vi "RealSense_HelloWorld_PointCloud.vi"() -> ()   [LabVIEW 2017]
doc: "Simple Demo showing how to connect a RealSense Camera to stream COLOR and DEPTH from the stereo camera of a D4xx series camera."
uses:
  libRealSense3.lvlib
  <vilib>/picture/3D Picture Control/NI_3D Picture Control.lvlib
  <vilib>/Utility/miscctls.llb/LV3DPointTypeDef.ctl
  <vilib>/Utility/miscctls.llb/LVRGBAColorTypeDef.ctl
  <vilib>/picture/3D Picture Control/Object/Create Object (name).vi
panel:
  in  "stop and exit":bool
  in  "Color format":enum16{"Monochrome", "RGB internal (RGB)"}(ring)=enum."RGB internal (RGB)"
  in  "Display tab":T1(tab)
  out "Stream selection":u16(ring) items=["Depth + Left Color", "Unrectified L + R", "Rectified L + R", "Depth Only", "RGB ext. Only", "Depth + L Monochrome"]
  out "Found \nRealSense":bool=TRUE
  out "height":i32=720
  out "width":i32=1280
  out "init results":T2={"camera name"="Intel RealSense D415", "camera S/N"="725112060291", "F/W"="05.12.01.00", "Sensor name"="Stereo Module", "api_version"=23201, "rscontext"=2279652045952, "device_list"=2279390748064, "device count"=1, "Dev out"=2279652602464, "sensor_list"=2279759543328, "sensor count"=2, "Sensor out"=2279397784752}
  in  "Select Resolution":u16(ring)=32 items=["424 x 240 @6fps", "424 x 240 @15fps", "424 x 240 @30fps", "424 x 240 @60fps", "424 x 240 @90fps", "480 x 270 @6fps", "480 x 270 @15fps", "480 x 270 @30fps", "480 x 270 @60fps", "480 x 270 @90fps", "640 x 360 @6fps", "640 x 360 @15fps", "640 x 360 @30fps", "640 x 360 @60fps", "640 x 360 @90fps", "640 x 480 @6fps", "640 x 480 @15fps", "640 x 480 @30fps", "640 x 480 @60fps", "640 x 480 @90fps", "848 x 100 @6fps", "848 x 100 @15fps", "848 x 100 @30fps", "848 x 100 @60fps", "848 x 100 @90fps", "848 x 480 @6fps", "848 x 480 @15fps", "848 x 480 @30fps", "848 x 480 @60fps", "848 x 480 @90fps", "1280 x 720 @6fps", "1280 x 720 @15fps", "1280 x 720 @30fps", "1280 x 720 @60fps"]
  in  "Sensor index":i32
  in  "Device index":i32
  out "L-R Baseline, mm":sgl=-54.83181
  out "fy":sgl=952.6064 format="%#_5g"
  out "fx":sgl=952.6064 format="%#_5g"
  out "ppy":sgl=370.69974 format="%#_5g"
  out "ppx":sgl=634.5728 format="%#_5g"
  in  "Exposure,us":sgl=33000.0
  in  "Autoexposure":bool=TRUE
  in  "Depth Presets":T3(ring)=enum."Face2"
  in  "Color Presets":T4(ring)=enum."DS410 (DS5a) 4"
  in  "Laser on/off":bool=TRUE
  in  "Gain(16-248)":sgl=16.0 min=16 max=248
  in  "Update Presets":bool
  in  "Laser \nPower (mW)":dbl(slide)=155.72448 min=0.0 max=360.0 scale=0.36..360.0
  in  "Range Scale":enum16{"200m", "100m", "60m", "6m", "2m", "1m"}(ring)=enum."6m"
  out "RGB image":picture
  out "Depth map":sgl[][](graph)
  out "3D Picture":refnum<vi>(3d-picture)
  out "init error":string="\rNo Error\rNo Error\rNo Error\rNo Error\rNo Error\rNo Error\rNo Error\r\rNo Error\rNo Error"
  out "Capture2 error":string="No Error"
  out "Start Error":string="No Error\rNo Error\rNo Error"
  out "Config error":string="No Error\rNo Error"
  out "Capture1 Error":string="No Error"
  out "Close Error":string="No Error\rNo Error\rNo Error\rNo Error"
  out "release frame error":string="No Error"
  out "iteration":i32=187
  in  "stop":bool=TRUE
  # "RealSense Hello World: PointCloud"
  # "This demo shows how to connect a RealSense D4xx(e) Depth Camera, and display the textured PointCloud."
  # "Note; When you change Depth Preset you need to stop and restart for the HDAD settings to take effect.\n\nTry the Color preset called \"Remove IR2\". It will remove the laser projector from the RGB 1280x720 image."
  # "INTRINSICS & EXTRINSICS"
  # "SELECT THE RESOLUTION"
  # "Recommendation:\nFor D435: 848x480, D415: 1280x720"
  # "COLOR / LEFT MONO"
  # "DEPTH MAP"
  # "Changes Color scale for Depth Map."
  # "20-1660000"
  # "3D POINTCLOUD"
  # "Rotate: Drag image\nMove X-Y: HOLD DOWN CTRL while dragging.\nZoom: SHIFT while dragging."
  # "ERRORS"
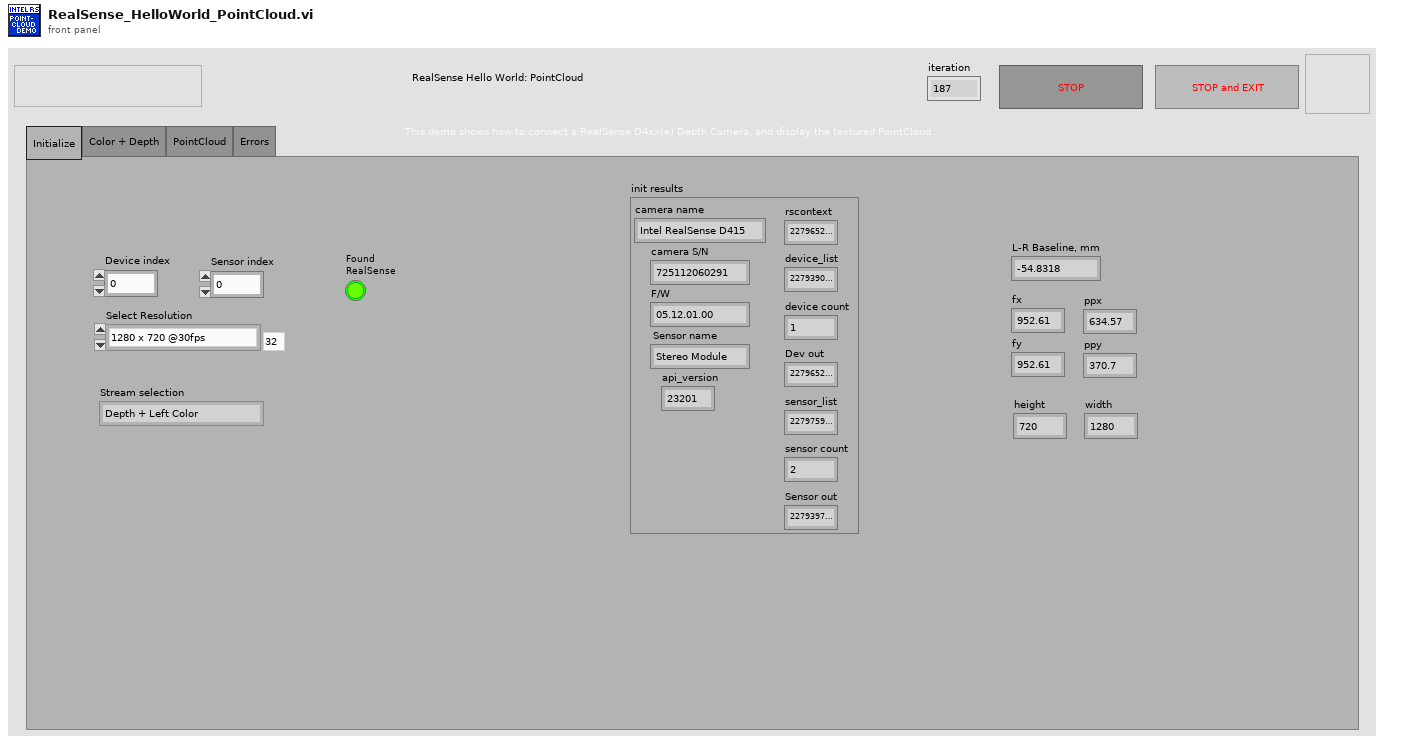
[diagram p1: front panel]
types:
  T1 = enum32{"Initialize", "Color + Depth", "PointCloud", "Errors"}
  T2 = cluster{"camera name":string, "camera S/N":string, "F/W":string, "Sensor name":string, "api_version":i32, "rscontext":u64, "device_list":u64, "device count":i32, "Dev out":u64, "sensor_list":u64, "sensor count":i32, "Sensor out":u64}
  T3 = enum16{"Custom", "Original", "New Depth 1", "New Depth 2", "Depth Active 1", "Active 3D Scan", "Active Short A", "Active Short C", "Face", "Face2", "Best Box", "High Density", "Medium Density", "High Accuracy", "Hand", "Short Range", "Flat wall", "Load .JSON", "Load .JSON2"}
  T4 = enum16{"Custom", "RS400 (DS5p)", "RS400 (DS5p) 2", "RS400 (DS5p) 3", "RS400 (DS5p) 4", "RS400 (DS5p) 5", "RS410 (DS5a)", "RS410 (DS5a) 2", "DS410 (DS5a) 3", "DS410 (DS5a) 4", "DS410+IR", "DS5LR", "DS5LR-2", "DS5LR no pattern", "RS410 Remove IR", "RS410 Remove IR 2", "DS5micro", "D435"}
  T5 = cluster{"width":i32, "height":i32, "fps":i32, "Profile":u64, "ppx":sgl, "ppy":sgl, "fx":sgl, "fy":sgl, "model":u32}
  T6 = enum16{"Overall", "Per Primitive", "Per Vertex", "Binding Off"}
  T7 = enum16{"Points", "Lines", "Line Strip", "Line Loop", "Triangles", "Triangle Strip", "Triangle Fan", "Quads", "Quad Strip", "Polygon"}
  T8 = enum16{"Depth", "Color (ext.)", "Color (left) ", "IR Left", "IR Right", "IR Left (Y16)", "IR Right (Y16)"}
  T9 = cluster{"R":dbl, "G":dbl, "B":dbl, "Alpha":dbl}[]
  T10 = typedef "LVRGBAColorTypeDef.ctl" = cluster{"Red":sgl, "Green":sgl, "Blue":sgl, "Alpha":sgl}
  T11 = typedef "LV3DPointTypeDef.ctl" = cluster{"X":sgl, "Y":sgl, "Z":sgl}
  T12 = cluster{"Alpha":sgl, "Blue":sgl, "Green":sgl, "Red":sgl}
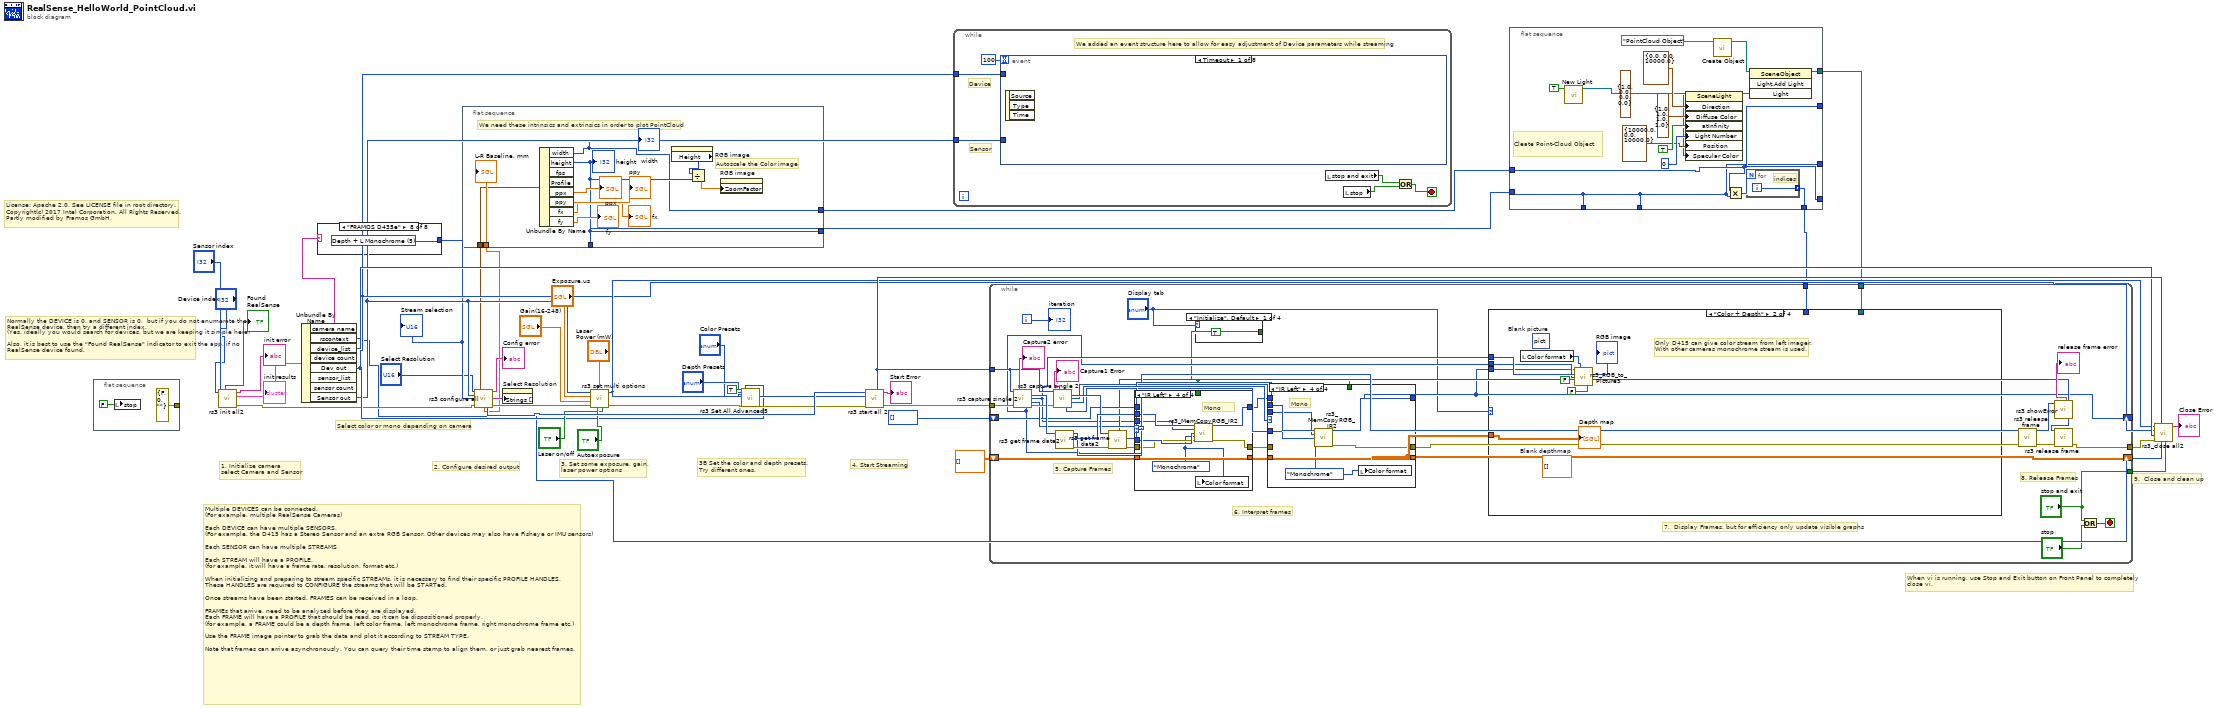
[diagram p0: block diagram]
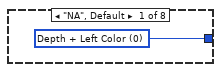
[diagram p2: hidden frame]
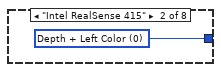
[diagram p3: hidden frame]
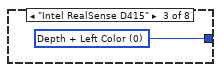
[diagram p4: hidden frame]
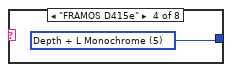
[diagram p5: hidden frame]
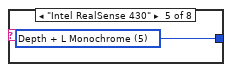
[diagram p6: hidden frame]
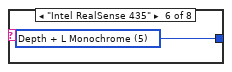
[diagram p7: hidden frame]
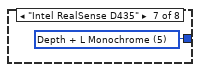
[diagram p8: hidden frame]
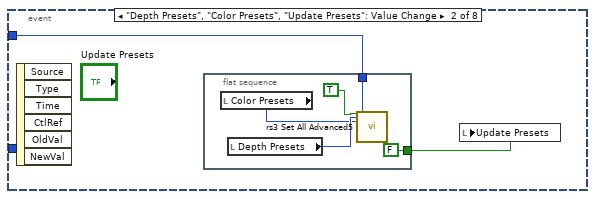
[diagram p9: hidden frame]
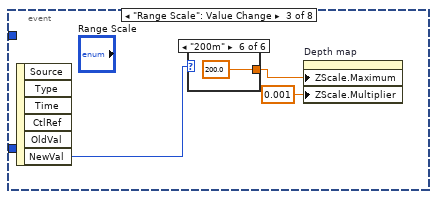
[diagram p10: hidden frame]
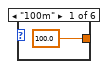
[diagram p11: hidden frame]
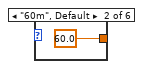
[diagram p12: hidden frame]
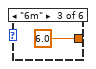
[diagram p13: hidden frame]
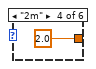
[diagram p14: hidden frame]
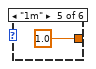
[diagram p15: hidden frame]
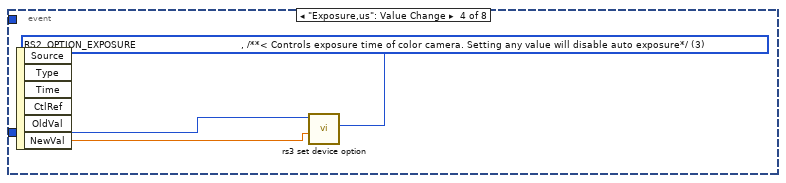
[diagram p16: hidden frame]
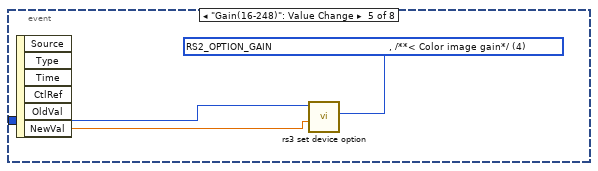
[diagram p17: hidden frame]
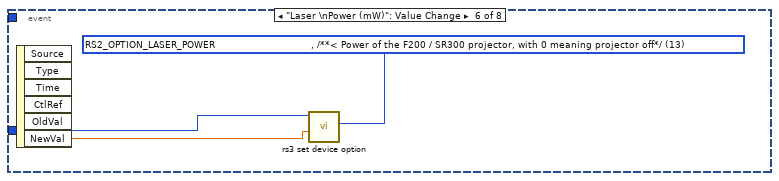
[diagram p18: hidden frame]
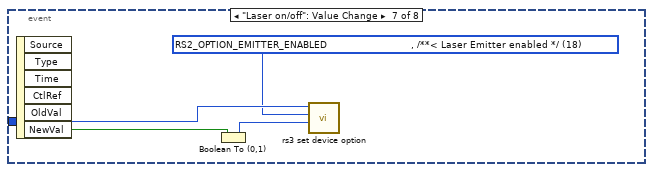
[diagram p19: hidden frame]
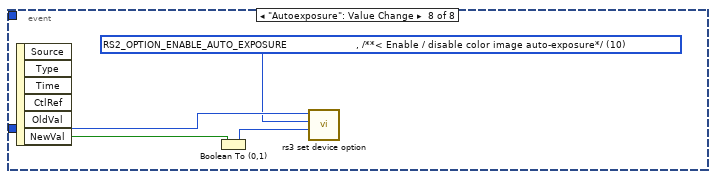
[diagram p20: hidden frame]
diagram:
  # "When vi is running, use Stop and Exit button on Front Panel to completely\nclose vi."
  # "License: Apache 2.0. See LICENSE file in root directory.\nCopyright(c) 2017 Intel Corporation. All Rights Reserved.\nPartly modified by Framos GmbH."
  # "3B Set the color and depth presets.\nTry different ones."
  # "Select color or mono depending on camera"
  # "Normally the DEVICE is 0, and SENSOR is 0,  but if you do not enumerate the RealSense device, then try a different index.\n(Yes, ideally you would search for devices, but we are keeping it simple here)\n\nAlso, it is best to use the \"Found RealSense\" indicator to exit the app, if no RealSense device found."
  # "Multiple DEVICES can be connected. \n(For example, multiple RealSense Cameras)\n\nEach DEVICE can have multiple SENSORS. \n(For example, the D415 has a Stereo Sensor and an extra RGB Sensor. Other devices may also have Fisheye or IMU sensors) \n\nEach SENSOR can have multiple STREAMS\n\nEach STREAM will have a PROFILE. \n(for example, it will have a frame rate, resolution, format etc.)\n\nWhen initializing and preparing to stream specific STREAMs, it is necessary to find their specific PROFILE HANDLES.\nThese HANDLES are required to CONFIGURE the streams that will be STARTed. \n\nOnce streams have been started, FRAMES can be received in a loop. \n \nFRAMEs that arrive, need to be analyzed before they are displayed. \nEach FRAME will have a PROFILE that should be read, so it can be dispositioned properly.\n(for example, a FRAME could be a depth frame, left color frame, left monochrome frame, right monochrome frame etc.)\n\nUse the FRAME image pointer to grab the data and plot it according to STREAM TYPE.\n\nNote that frames can arrive asynchronously. You can query their time stamp to align them, or just grab nearest frames."
  # "9.  Close and clean up"
  # "4. Start Streaming"
  # "3. Set some exposure, gain, \nlaser power options"
  # "2. Configure desired output"
  # "1. Initialize camera\nselect Camera and Sensor"
  n1 = flat-sequence {
    tunnel: [errorcluster {"status"=FALSE, "code"=0, "source"=""} ("error in")] -> _
    frame #0 {
      n2 = local write "stop"(FALSE ("stop")) -> ()
    }
  }
  n3 = call "rs3 init all2.vi"("Select Device"="Device index", "Select Sensor"="Sensor index") -> ("error out"=w9:errorcluster, "init results"=w14:T2, "init error"=→"init error":string, "Found RealSense"=→"Found \nRealSense":bool)  [unwired: 3 in, 3 out]
  "init results" <- w14
  n4 = Unbundle By Name(w14) -> ("camera name"=w8:string, "rscontext"=w6:u64, "device_list"=w37:u64, "Dev out"=w21:u64, "Sensor out"=w20:u64)  [unwired: 3 out]
  n5 = case shown="\"FRAMOS D435e\"" w8 {
    tunnel: [w45 w46 w47 w48 w49 w50 w51 w52] -> w7
    frame "NA", Default {
      w45 = u16 0 items=["Depth + Left Color", "Unrectified L + R", "Rectified L + R", "Depth Only", "RGB ext. Only", "Depth + L Monochrome"] ("Stream selection")
    }
    frame "Intel RealSense 415" {
      w46 = u16 0 items=["Depth + Left Color", "Unrectified L + R", "Rectified L + R", "Depth Only", "RGB ext. Only", "Depth + L Monochrome"] ("Stream selection")
    }
    frame "Intel RealSense D415" {
      w47 = u16 0 items=["Depth + Left Color", "Unrectified L + R", "Rectified L + R", "Depth Only", "RGB ext. Only", "Depth + L Monochrome"] ("Stream selection")
    }
    frame "FRAMOS D415e" {
      w48 = u16 5 items=["Depth + Left Color", "Unrectified L + R", "Rectified L + R", "Depth Only", "RGB ext. Only", "Depth + L Monochrome"] ("Stream selection")
    }
    frame "Intel RealSense 430" {
      w49 = u16 5 items=["Depth + Left Color", "Unrectified L + R", "Rectified L + R", "Depth Only", "RGB ext. Only", "Depth + L Monochrome"] ("Stream selection")
    }
    frame "Intel RealSense 435" {
      w50 = u16 5 items=["Depth + Left Color", "Unrectified L + R", "Rectified L + R", "Depth Only", "RGB ext. Only", "Depth + L Monochrome"] ("Stream selection")
    }
    frame "Intel RealSense D435" {
      w51 = u16 5 items=["Depth + Left Color", "Unrectified L + R", "Rectified L + R", "Depth Only", "RGB ext. Only", "Depth + L Monochrome"] ("Stream selection")
    }
    frame "FRAMOS D435e" {
      w52 = u16 5 items=["Depth + Left Color", "Unrectified L + R", "Rectified L + R", "Depth Only", "RGB ext. Only", "Depth + L Monochrome"] ("Stream selection")
    }
  }
  "Stream selection" <- w7
  n6 = flat-sequence {
    tunnel: w18 -> [w62]
    tunnel: w17 -> [w61]
    tunnel: [w54] -> _
    tunnel: [w53] -> w4
    tunnel: [w54] -> w3
    frame #0 {
      # "Autoscale the Color image"
      # "We need these intrinsics and extrinsics in order to plot PointCloud"
      n7 = Unbundle By Name(w61) -> ("width"=w53:i32, "height"=w54:i32, "ppx"=→"ppx":sgl, "ppy"=→"ppy":sgl, "fx"=→"fx":sgl, "fy"=→"fy":sgl)  [unwired: 2 out]
      "height" <- w54
      "width" <- w53
      n8 = property on="RGB image" class="Pict"() -> ("Height"=w60:u32)  [unwired: 2 in, 2 out]
      n9 = Divide(x=w60, y=w54) -> (x/y=w59:dbl)
      n10 = property on="RGB image" class="Pict"("ZoomFactor"=w59) -> ()  [unwired: 2 in, 2 out]
      "L-R Baseline, mm" <- w62
    }
  }
  n11 = call "rs3 configure all.vi"("Select Resolution"="Select Resolution", "Sensor in"=w20, "Stream selection"=w7, "error in (no error)"=w9) -> ("Output stream L"=w17:T5, "config error"=→"Config error":string, "Output stream"=w34:string[], "L-R Baseline, mm"=w18:sgl, "Stream Profile Handles"=w42:u64[], "error out"=w33:errorcluster)  [unwired: 2 in, 4 out]
  n12 = property on="Select Resolution" class="Ring (strict)"("Strings []"=w34) -> ()  [unwired: 2 in, 2 out]
  n13 = call "rs3 set multi options.vi"("laser on/off"="Laser on/off", "autoexposure"="Autoexposure", "Laser power, mW (0-360)"="Laser \nPower (mW)", "error in (no error)"=w33, "Gain(16-248)"="Gain(16-248)", "Exposure, us"="Exposure,us", "Sensor in"=w20) -> ("error out"=w26:errorcluster, "Sensor out"=w32:u64)  [unwired: 2 in, 1 out]
  n14 = call "rs3 Set All Advanced5.vi"("Set Color Corr"=TRUE, "Depth Presets"="Depth Presets", "Color Presets"="Color Presets", "error in (no error)"=w26, "device in"=w21) -> ("error out"=w25:errorcluster)  [unwired: 20 in, 2 out]
  n15 = call "rs3 start all 2.vi"("error in (no error)"=w25, "Sensor in"=w32, "Stream profile array"=w42) -> ("error out"=w35:errorcluster, "Config Error"=→"Start Error":string, "queue out"=w41:u64)  [unwired: 5 in, 1 out]
  n16 = while {
    tunnel: w21 -> [w68]
    tunnel: w20 -> [w67]
    stop <- w63 stop-if-true
    # "Sensor"
    # "Device"
    # "We added an event structure here to allow for easy adjustment of Device parameters while streaming"
    n17 = event shown="[0] Timeout" {
      selector: _ -> [_ _ _ _ _ _ _ _]
      dyn-events: _ -> [_ _ _ _ _ _ _ _]
      timeout: 100 -> [_ _ _ _ _ _ _ _]
      tunnel: w68 -> [_ w70 _ _ _ _ _ _]
      tunnel: w67 -> [_ _ _ w87 w90 w93 w97 w101]
      event Timeout {
        n18 = event-data() -> ()  [unwired: 1 in, 3 out]
      }
      event "Depth Presets", "Color Presets", "Update Presets": Value Change {
        n19 = event-data() -> ()  [unwired: 1 in, 6 out]
        n20 = flat-sequence {
          tunnel: w70 -> [w72]
          tunnel: [FALSE ("Update Presets")] -> w69
          frame #0 {
            n21 = local read "Color Presets"() -> (w74:T4)
            n22 = local read "Depth Presets"() -> (w75:T3)
            n23 = call "rs3 Set All Advanced5.vi"("Set Color Corr"=TRUE, "Depth Presets"=w75, "Color Presets"=w74, "device in"=w72) -> ()  [unwired: 21 in, 3 out]
          }
        }
        n24 = local write "Update Presets"(w69) -> ()
      }
      event "Range Scale": Value Change {
        n25 = event-data() -> ("NewVal"=w77:enum16{"200m", "100m", "60m", "6m", "2m", "1m"})  [unwired: 1 in, 5 out]
        n26 = case shown="\"200m\"" w77 {
          tunnel: [100.0 ("Z Scale.Offset and Multiplier:Multiplier") 60.0 ("Z Scale.Offset and Multiplier:Multiplier") 6.0 ("Z Scale.Offset and Multiplier:Multiplier") 2.0 ("Z Scale.Offset and Multiplier:Multiplier") 1.0 ("Z Scale.Offset and Multiplier:Multiplier") 200.0 ("Z Scale.Offset and Multiplier:Multiplier")] -> w76
          frame "100m" {
          }
          frame "60m", Default {
          }
          frame "6m" {
          }
          frame "2m" {
          }
          frame "1m" {
          }
          frame "200m" {
          }
        }
        n27 = property on="Depth map" class="IntGraph (strict)"("ZScale.Maximum"=w76, "ZScale.Multiplier"=0.001 ("Z Scale.Offset and Multiplier:Multiplier")) -> ()  [unwired: 2 in, 2 out]
      }
      event "Exposure,us": Value Change {
        w85 = u16 3 items=["    RS2_OPTION_BACKLIGHT_COMPENSATION                     , /**< Enable / disable color backlight compensation*/", "    RS2_OPTION_BRIGHTNESS                                 , /**< Color image brightness*/", "    RS2_OPTION_CONTRAST                                   , /**< Color image contrast*/", "    RS2_OPTION_EXPOSURE                                   , /**< Controls exposure time of color camera. Setting any value will disable auto exposure*/", "    RS2_OPTION_GAIN                                       , /**< Color image gain*/", "    RS2_OPTION_GAMMA                                      , /**< Color image gamma setting*/", "    RS2_OPTION_HUE                                        , /**< Color image hue*/", "    RS2_OPTION_SATURATION                                 , /**< Color image saturation setting*/", "    RS2_OPTION_SHARPNESS                                  , /**< Color image sharpness setting*/", "    RS2_OPTION_WHITE_BALANCE                              , /**< Controls white balance of color image. Setting any value will disable auto white balance*/", "    RS2_OPTION_ENABLE_AUTO_EXPOSURE                       , /**< Enable / disable color image auto-exposure*/", "    RS2_OPTION_ENABLE_AUTO_WHITE_BALANCE                  , /**< Enable / disable color image auto-white-balance*/", "    RS2_OPTION_VISUAL_PRESET                              , /**< Provide access to several recommend sets of option presets for the depth camera */", "    RS2_OPTION_LASER_POWER                                , /**< Power of the F200 / SR300 projector, with 0 meaning projector off*/", "    RS2_OPTION_ACCURACY                                   , /**< Set the number of patterns projected per frame. The higher the accuracy value the more patterns projected. Increasing the number of patterns help to achieve better accuracy. Note that this c", "    RS2_OPTION_MOTION_RANGE                               , /**< Motion vs. Range trade-off, with lower values allowing for better motion sensitivity and higher values allowing for better depth range*/", "    RS2_OPTION_FILTER_OPTION                              , /**< Set the filter to apply to each depth frame. Each one of the filter is optimized per the application requirements*/", "    RS2_OPTION_CONFIDENCE_THRESHOLD                       , /**< The confidence level threshold used by the Depth algorithm pipe to set whether a pixel will get a valid range or will be marked with invalid range*/", "    RS2_OPTION_EMITTER_ENABLED                            , /**< Laser Emitter enabled */", "    RS2_OPTION_FRAMES_QUEUE_SIZE                          , /**< Number of frames the user is allowed to keep per stream. Trying to hold-on to more frames will cause frame-drops.*/", "    RS2_OPTION_TOTAL_FRAME_DROPS                          , /**< Total number of detected frame drops from all streams */", "    RS2_OPTION_AUTO_EXPOSURE_MODE                         , /**< Auto-Exposure modes: Static, Anti-Flicker and Hybrid */", "    RS2_OPTION_POWER_LINE_FREQUENCY                       , /**< Power Line Frequency control for anti-flickering Off/50Hz/60Hz/Auto */", "    RS2_OPTION_ASIC_TEMPERATURE                           , /**< Current Asic Temperature */", "    RS2_OPTION_ERROR_POLLING_ENABLED                      , /**< disable error handling */", "    RS2_OPTION_PROJECTOR_TEMPERATURE                      , /**< Current Projector Temperature */", "    RS2_OPTION_OUTPUT_TRIGGER_ENABLED                     , /**< Enable / disable trigger to be outputed from the camera to any external device on every depth frame */", "    RS2_OPTION_MOTION_MODULE_TEMPERATURE                  , /**< Current Motion-Module Temperature */", "    RS2_OPTION_DEPTH_UNITS                                , /**< Number of meters represented by a single depth unit */", "    RS2_OPTION_ENABLE_MOTION_CORRECTION                   , /**< Enable/Disable automatic correction of the motion data */", "    RS2_OPTION_AUTO_EXPOSURE_PRIORITY                     , /**< Allows sensor to dynamically ajust the frame rate depending on lighting conditions */", "    RS2_OPTION_COUNT                                      , /**< Number of enumeration values. Not a valid input: intended to be used in for-loops. */"] ("RS Option")
        n28 = event-data() -> ("NewVal"=w86:sgl)  [unwired: 1 in, 5 out]
        n29 = call "rs3 set device option.vi"("value"=w86, "RS Option"=w85, "Sensor in"=w87) -> ()  [unwired: 6 in, 3 out]
      }
      event "Gain(16-248)": Value Change {
        w88 = u16 4 items=["    RS2_OPTION_BACKLIGHT_COMPENSATION                     , /**< Enable / disable color backlight compensation*/", "    RS2_OPTION_BRIGHTNESS                                 , /**< Color image brightness*/", "    RS2_OPTION_CONTRAST                                   , /**< Color image contrast*/", "    RS2_OPTION_EXPOSURE                                   , /**< Controls exposure time of color camera. Setting any value will disable auto exposure*/", "    RS2_OPTION_GAIN                                       , /**< Color image gain*/", "    RS2_OPTION_GAMMA                                      , /**< Color image gamma setting*/", "    RS2_OPTION_HUE                                        , /**< Color image hue*/", "    RS2_OPTION_SATURATION                                 , /**< Color image saturation setting*/", "    RS2_OPTION_SHARPNESS                                  , /**< Color image sharpness setting*/", "    RS2_OPTION_WHITE_BALANCE                              , /**< Controls white balance of color image. Setting any value will disable auto white balance*/", "    RS2_OPTION_ENABLE_AUTO_EXPOSURE                       , /**< Enable / disable color image auto-exposure*/", "    RS2_OPTION_ENABLE_AUTO_WHITE_BALANCE                  , /**< Enable / disable color image auto-white-balance*/", "    RS2_OPTION_VISUAL_PRESET                              , /**< Provide access to several recommend sets of option presets for the depth camera */", "    RS2_OPTION_LASER_POWER                                , /**< Power of the F200 / SR300 projector, with 0 meaning projector off*/", "    RS2_OPTION_ACCURACY                                   , /**< Set the number of patterns projected per frame. The higher the accuracy value the more patterns projected. Increasing the number of patterns help to achieve better accuracy. Note that this c", "    RS2_OPTION_MOTION_RANGE                               , /**< Motion vs. Range trade-off, with lower values allowing for better motion sensitivity and higher values allowing for better depth range*/", "    RS2_OPTION_FILTER_OPTION                              , /**< Set the filter to apply to each depth frame. Each one of the filter is optimized per the application requirements*/", "    RS2_OPTION_CONFIDENCE_THRESHOLD                       , /**< The confidence level threshold used by the Depth algorithm pipe to set whether a pixel will get a valid range or will be marked with invalid range*/", "    RS2_OPTION_EMITTER_ENABLED                            , /**< Laser Emitter enabled */", "    RS2_OPTION_FRAMES_QUEUE_SIZE                          , /**< Number of frames the user is allowed to keep per stream. Trying to hold-on to more frames will cause frame-drops.*/", "    RS2_OPTION_TOTAL_FRAME_DROPS                          , /**< Total number of detected frame drops from all streams */", "    RS2_OPTION_AUTO_EXPOSURE_MODE                         , /**< Auto-Exposure modes: Static, Anti-Flicker and Hybrid */", "    RS2_OPTION_POWER_LINE_FREQUENCY                       , /**< Power Line Frequency control for anti-flickering Off/50Hz/60Hz/Auto */", "    RS2_OPTION_ASIC_TEMPERATURE                           , /**< Current Asic Temperature */", "    RS2_OPTION_ERROR_POLLING_ENABLED                      , /**< disable error handling */", "    RS2_OPTION_PROJECTOR_TEMPERATURE                      , /**< Current Projector Temperature */", "    RS2_OPTION_OUTPUT_TRIGGER_ENABLED                     , /**< Enable / disable trigger to be outputed from the camera to any external device on every depth frame */", "    RS2_OPTION_MOTION_MODULE_TEMPERATURE                  , /**< Current Motion-Module Temperature */", "    RS2_OPTION_DEPTH_UNITS                                , /**< Number of meters represented by a single depth unit */", "    RS2_OPTION_ENABLE_MOTION_CORRECTION                   , /**< Enable/Disable automatic correction of the motion data */", "    RS2_OPTION_AUTO_EXPOSURE_PRIORITY                     , /**< Allows sensor to dynamically ajust the frame rate depending on lighting conditions */", "    RS2_OPTION_COUNT                                      , /**< Number of enumeration values. Not a valid input: intended to be used in for-loops. */"] ("RS Option")
        n30 = event-data() -> ("NewVal"=w89:sgl)  [unwired: 1 in, 5 out]
        n31 = call "rs3 set device option.vi"("value"=w89, "RS Option"=w88, "Sensor in"=w90) -> ()  [unwired: 6 in, 3 out]
      }
      event "Laser \nPower (mW)": Value Change {
        w91 = u16 13 items=["    RS2_OPTION_BACKLIGHT_COMPENSATION                     , /**< Enable / disable color backlight compensation*/", "    RS2_OPTION_BRIGHTNESS                                 , /**< Color image brightness*/", "    RS2_OPTION_CONTRAST                                   , /**< Color image contrast*/", "    RS2_OPTION_EXPOSURE                                   , /**< Controls exposure time of color camera. Setting any value will disable auto exposure*/", "    RS2_OPTION_GAIN                                       , /**< Color image gain*/", "    RS2_OPTION_GAMMA                                      , /**< Color image gamma setting*/", "    RS2_OPTION_HUE                                        , /**< Color image hue*/", "    RS2_OPTION_SATURATION                                 , /**< Color image saturation setting*/", "    RS2_OPTION_SHARPNESS                                  , /**< Color image sharpness setting*/", "    RS2_OPTION_WHITE_BALANCE                              , /**< Controls white balance of color image. Setting any value will disable auto white balance*/", "    RS2_OPTION_ENABLE_AUTO_EXPOSURE                       , /**< Enable / disable color image auto-exposure*/", "    RS2_OPTION_ENABLE_AUTO_WHITE_BALANCE                  , /**< Enable / disable color image auto-white-balance*/", "    RS2_OPTION_VISUAL_PRESET                              , /**< Provide access to several recommend sets of option presets for the depth camera */", "    RS2_OPTION_LASER_POWER                                , /**< Power of the F200 / SR300 projector, with 0 meaning projector off*/", "    RS2_OPTION_ACCURACY                                   , /**< Set the number of patterns projected per frame. The higher the accuracy value the more patterns projected. Increasing the number of patterns help to achieve better accuracy. Note that this c", "    RS2_OPTION_MOTION_RANGE                               , /**< Motion vs. Range trade-off, with lower values allowing for better motion sensitivity and higher values allowing for better depth range*/", "    RS2_OPTION_FILTER_OPTION                              , /**< Set the filter to apply to each depth frame. Each one of the filter is optimized per the application requirements*/", "    RS2_OPTION_CONFIDENCE_THRESHOLD                       , /**< The confidence level threshold used by the Depth algorithm pipe to set whether a pixel will get a valid range or will be marked with invalid range*/", "    RS2_OPTION_EMITTER_ENABLED                            , /**< Laser Emitter enabled */", "    RS2_OPTION_FRAMES_QUEUE_SIZE                          , /**< Number of frames the user is allowed to keep per stream. Trying to hold-on to more frames will cause frame-drops.*/", "    RS2_OPTION_TOTAL_FRAME_DROPS                          , /**< Total number of detected frame drops from all streams */", "    RS2_OPTION_AUTO_EXPOSURE_MODE                         , /**< Auto-Exposure modes: Static, Anti-Flicker and Hybrid */", "    RS2_OPTION_POWER_LINE_FREQUENCY                       , /**< Power Line Frequency control for anti-flickering Off/50Hz/60Hz/Auto */", "    RS2_OPTION_ASIC_TEMPERATURE                           , /**< Current Asic Temperature */", "    RS2_OPTION_ERROR_POLLING_ENABLED                      , /**< disable error handling */", "    RS2_OPTION_PROJECTOR_TEMPERATURE                      , /**< Current Projector Temperature */", "    RS2_OPTION_OUTPUT_TRIGGER_ENABLED                     , /**< Enable / disable trigger to be outputed from the camera to any external device on every depth frame */", "    RS2_OPTION_MOTION_MODULE_TEMPERATURE                  , /**< Current Motion-Module Temperature */", "    RS2_OPTION_DEPTH_UNITS                                , /**< Number of meters represented by a single depth unit */", "    RS2_OPTION_ENABLE_MOTION_CORRECTION                   , /**< Enable/Disable automatic correction of the motion data */", "    RS2_OPTION_AUTO_EXPOSURE_PRIORITY                     , /**< Allows sensor to dynamically ajust the frame rate depending on lighting conditions */", "    RS2_OPTION_COUNT                                      , /**< Number of enumeration values. Not a valid input: intended to be used in for-loops. */"] ("RS Option")
        n32 = event-data() -> ("NewVal"=w92:dbl)  [unwired: 1 in, 5 out]
        n33 = call "rs3 set device option.vi"("value"=w92, "RS Option"=w91, "Sensor in"=w93) -> ()  [unwired: 6 in, 3 out]
      }
      event "Laser on/off": Value Change {
        w96 = u16 18 items=["    RS2_OPTION_BACKLIGHT_COMPENSATION                     , /**< Enable / disable color backlight compensation*/", "    RS2_OPTION_BRIGHTNESS                                 , /**< Color image brightness*/", "    RS2_OPTION_CONTRAST                                   , /**< Color image contrast*/", "    RS2_OPTION_EXPOSURE                                   , /**< Controls exposure time of color camera. Setting any value will disable auto exposure*/", "    RS2_OPTION_GAIN                                       , /**< Color image gain*/", "    RS2_OPTION_GAMMA                                      , /**< Color image gamma setting*/", "    RS2_OPTION_HUE                                        , /**< Color image hue*/", "    RS2_OPTION_SATURATION                                 , /**< Color image saturation setting*/", "    RS2_OPTION_SHARPNESS                                  , /**< Color image sharpness setting*/", "    RS2_OPTION_WHITE_BALANCE                              , /**< Controls white balance of color image. Setting any value will disable auto white balance*/", "    RS2_OPTION_ENABLE_AUTO_EXPOSURE                       , /**< Enable / disable color image auto-exposure*/", "    RS2_OPTION_ENABLE_AUTO_WHITE_BALANCE                  , /**< Enable / disable color image auto-white-balance*/", "    RS2_OPTION_VISUAL_PRESET                              , /**< Provide access to several recommend sets of option presets for the depth camera */", "    RS2_OPTION_LASER_POWER                                , /**< Power of the F200 / SR300 projector, with 0 meaning projector off*/", "    RS2_OPTION_ACCURACY                                   , /**< Set the number of patterns projected per frame. The higher the accuracy value the more patterns projected. Increasing the number of patterns help to achieve better accuracy. Note that this c", "    RS2_OPTION_MOTION_RANGE                               , /**< Motion vs. Range trade-off, with lower values allowing for better motion sensitivity and higher values allowing for better depth range*/", "    RS2_OPTION_FILTER_OPTION                              , /**< Set the filter to apply to each depth frame. Each one of the filter is optimized per the application requirements*/", "    RS2_OPTION_CONFIDENCE_THRESHOLD                       , /**< The confidence level threshold used by the Depth algorithm pipe to set whether a pixel will get a valid range or will be marked with invalid range*/", "    RS2_OPTION_EMITTER_ENABLED                            , /**< Laser Emitter enabled */", "    RS2_OPTION_FRAMES_QUEUE_SIZE                          , /**< Number of frames the user is allowed to keep per stream. Trying to hold-on to more frames will cause frame-drops.*/", "    RS2_OPTION_TOTAL_FRAME_DROPS                          , /**< Total number of detected frame drops from all streams */", "    RS2_OPTION_AUTO_EXPOSURE_MODE                         , /**< Auto-Exposure modes: Static, Anti-Flicker and Hybrid */", "    RS2_OPTION_POWER_LINE_FREQUENCY                       , /**< Power Line Frequency control for anti-flickering Off/50Hz/60Hz/Auto */", "    RS2_OPTION_ASIC_TEMPERATURE                           , /**< Current Asic Temperature */", "    RS2_OPTION_ERROR_POLLING_ENABLED                      , /**< disable error handling */", "    RS2_OPTION_PROJECTOR_TEMPERATURE                      , /**< Current Projector Temperature */", "    RS2_OPTION_OUTPUT_TRIGGER_ENABLED                     , /**< Enable / disable trigger to be outputed from the camera to any external device on every depth frame */", "    RS2_OPTION_MOTION_MODULE_TEMPERATURE                  , /**< Current Motion-Module Temperature */", "    RS2_OPTION_DEPTH_UNITS                                , /**< Number of meters represented by a single depth unit */", "    RS2_OPTION_ENABLE_MOTION_CORRECTION                   , /**< Enable/Disable automatic correction of the motion data */", "    RS2_OPTION_AUTO_EXPOSURE_PRIORITY                     , /**< Allows sensor to dynamically ajust the frame rate depending on lighting conditions */", "    RS2_OPTION_COUNT                                      , /**< Number of enumeration values. Not a valid input: intended to be used in for-loops. */"] ("RS Option")
        n34 = event-data() -> ("NewVal"=w95:bool)  [unwired: 1 in, 5 out]
        n35 = Boolean To (0,1)(Boolean=w95) -> (0, 1=w94:i16)
        n36 = call "rs3 set device option.vi"("value"=w94, "RS Option"=w96, "Sensor in"=w97) -> ()  [unwired: 6 in, 3 out]
      }
      event "Autoexposure": Value Change {
        w100 = u16 10 items=["    RS2_OPTION_BACKLIGHT_COMPENSATION                     , /**< Enable / disable color backlight compensation*/", "    RS2_OPTION_BRIGHTNESS                                 , /**< Color image brightness*/", "    RS2_OPTION_CONTRAST                                   , /**< Color image contrast*/", "    RS2_OPTION_EXPOSURE                                   , /**< Controls exposure time of color camera. Setting any value will disable auto exposure*/", "    RS2_OPTION_GAIN                                       , /**< Color image gain*/", "    RS2_OPTION_GAMMA                                      , /**< Color image gamma setting*/", "    RS2_OPTION_HUE                                        , /**< Color image hue*/", "    RS2_OPTION_SATURATION                                 , /**< Color image saturation setting*/", "    RS2_OPTION_SHARPNESS                                  , /**< Color image sharpness setting*/", "    RS2_OPTION_WHITE_BALANCE                              , /**< Controls white balance of color image. Setting any value will disable auto white balance*/", "    RS2_OPTION_ENABLE_AUTO_EXPOSURE                       , /**< Enable / disable color image auto-exposure*/", "    RS2_OPTION_ENABLE_AUTO_WHITE_BALANCE                  , /**< Enable / disable color image auto-white-balance*/", "    RS2_OPTION_VISUAL_PRESET                              , /**< Provide access to several recommend sets of option presets for the depth camera */", "    RS2_OPTION_LASER_POWER                                , /**< Power of the F200 / SR300 projector, with 0 meaning projector off*/", "    RS2_OPTION_ACCURACY                                   , /**< Set the number of patterns projected per frame. The higher the accuracy value the more patterns projected. Increasing the number of patterns help to achieve better accuracy. Note that this c", "    RS2_OPTION_MOTION_RANGE                               , /**< Motion vs. Range trade-off, with lower values allowing for better motion sensitivity and higher values allowing for better depth range*/", "    RS2_OPTION_FILTER_OPTION                              , /**< Set the filter to apply to each depth frame. Each one of the filter is optimized per the application requirements*/", "    RS2_OPTION_CONFIDENCE_THRESHOLD                       , /**< The confidence level threshold used by the Depth algorithm pipe to set whether a pixel will get a valid range or will be marked with invalid range*/", "    RS2_OPTION_EMITTER_ENABLED                            , /**< Laser Emitter enabled */", "    RS2_OPTION_FRAMES_QUEUE_SIZE                          , /**< Number of frames the user is allowed to keep per stream. Trying to hold-on to more frames will cause frame-drops.*/", "    RS2_OPTION_TOTAL_FRAME_DROPS                          , /**< Total number of detected frame drops from all streams */", "    RS2_OPTION_AUTO_EXPOSURE_MODE                         , /**< Auto-Exposure modes: Static, Anti-Flicker and Hybrid */", "    RS2_OPTION_POWER_LINE_FREQUENCY                       , /**< Power Line Frequency control for anti-flickering Off/50Hz/60Hz/Auto */", "    RS2_OPTION_ASIC_TEMPERATURE                           , /**< Current Asic Temperature */", "    RS2_OPTION_ERROR_POLLING_ENABLED                      , /**< disable error handling */", "    RS2_OPTION_PROJECTOR_TEMPERATURE                      , /**< Current Projector Temperature */", "    RS2_OPTION_OUTPUT_TRIGGER_ENABLED                     , /**< Enable / disable trigger to be outputed from the camera to any external device on every depth frame */", "    RS2_OPTION_MOTION_MODULE_TEMPERATURE                  , /**< Current Motion-Module Temperature */", "    RS2_OPTION_DEPTH_UNITS                                , /**< Number of meters represented by a single depth unit */", "    RS2_OPTION_ENABLE_MOTION_CORRECTION                   , /**< Enable/Disable automatic correction of the motion data */", "    RS2_OPTION_AUTO_EXPOSURE_PRIORITY                     , /**< Allows sensor to dynamically ajust the frame rate depending on lighting conditions */", "    RS2_OPTION_COUNT                                      , /**< Number of enumeration values. Not a valid input: intended to be used in for-loops. */"] ("RS Option")
        n37 = event-data() -> ("NewVal"=w99:bool)  [unwired: 1 in, 5 out]
        n38 = Boolean To (0,1)(Boolean=w99) -> (0, 1=w98:i16)
        n39 = call "rs3 set device option.vi"("value"=w98, "RS Option"=w100, "Sensor in"=w101) -> ()  [unwired: 6 in, 3 out]
      }
    }
    n40 = local read "stop and exit"() -> (w64:bool)
    n41 = local read "stop"() -> (w65:bool)
    n42 = Or(x=w64, y=w65) -> (x .or. y?=w63:bool)
  }
  n43 = while {
    tunnel: w41 -> [w130]
    tunnel: w35 -> [w140]
    tunnel: [w135] -> w40
    shift-right: [w110] -> _
    shift-left: sgl[][] [] ("2D Array Output") -> [w118]
    shift-right: [w112] -> _
    shift-left: u8[] [] ("Output Array") -> [w116]
    tunnel: w16 -> [w108]
    tunnel: w2 -> [w107]
    tunnel: ["stop and exit"] -> w5
    i -> [w139]
    stop <- w104 stop-if-true
    # "8. Release Frames"
    # "7.  Display Frames, but for efficiency only update visible graphs"
    # "6. Interpret frames"
    # "5. Capture Frames"
    n44 = call "rs3 capture single 2.vi"("queue in"=w130, "error in (no error)"=w140) -> ("Capture Error"=→"Capture2 error":string, "frame out"=w138:u64, "width"=w111:i32, "Stream type"=w119:T8, "height"=w109:i32, "error out"=w131:errorcluster)  [unwired: 2 in, 6 out]
    n45 = call "rs3 capture single 2.vi"("queue in"=w130, "error in (no error)"=w131) -> ("Capture Error"=→"Capture1 Error":string, "frame out"=w128:u64, "width"=w121:i32, "Stream type"=w123:T8, "height"=w120:i32)  [unwired: 2 in, 7 out]
    n46 = call "rs3 get frame data2.vi"("frame in"=w138) -> ("error out"=w134:errorcluster, "image pointer out"=w137:u64, "Frame out"=w114:u64)  [unwired: 7 in, 1 out]
    n47 = call "rs3 get frame data2.vi"("error in (no error)"=w134, "frame in"=w128) -> ("error out"=w133:errorcluster, "image pointer out"=w122:u64, "Frame out"=w113:u64)  [unwired: 6 in, 1 out]
    n48 = case shown="\"Initialize\", Default" "Display tab" {
      tunnel: [TRUE ("Transpose") TRUE ("Transpose") FALSE ("Transpose") TRUE ("Transpose")] -> w105
      frame "Initialize", Default {
      }
      frame "Color + Depth" {
      }
      frame "PointCloud" {
      }
      frame "Errors" {
      }
    }
    n49 = case shown="\"IR Left\"" w119 {
      tunnel: [w217 w223 w231 w239] -> w125
      tunnel: w137 -> [_ w221 w234 w242]
      tunnel: w111 -> [_ w220 w233 w241]
      tunnel: w109 -> [_ w219 w232 w240]
      tunnel: w133 -> [w217 w224 w230 w238]
      tunnel: [w216 w225 w228 w236] -> w117
      tunnel: w118 -> [w216 _ w228 w236]
      tunnel: w116 -> [w215 w222 _ _]
      tunnel: [w215 w222 w229 w237] -> w115
      tunnel: w105 -> [_ w218 _ _]
      frame "Color (ext.)", Default {
      }
      frame "Depth" {
        w226 = u16 0 items=["Y16", "Y8"] ("Image format")
        # "Depth"
        n50 = call "rs3_MemCopyUINT16_3.vi"("Image format"=w226, "Transpose"=w218, "error in (no error)"=w224, "Depth Y"=w219, "Depth X"=w220, "Zimage pointer"=w221) -> ("error out"=w223:errorcluster, "2D Array Output"=w225:sgl[][])  [unwired: 2 in, 2 out]
      }
      frame "Color (left) " {
        w227 = enum16{"Monochrome", "RGB internal (RGB)"}."RGB internal (RGB)" ("Color format")
        # "Color"
        n51 = call "rs3_MemCopyRGB_IR2.vi"("Zimage pointer"=w234, "RGB  X, width"=w233, "RGB Y, height"=w232, "Color format"=w227, "error in (no error)"=w230) -> ("Output Array"=w229:u8[], "error out"=w231:errorcluster)  [unwired: 8 in, 1 out]
        n52 = local write "Color format"(w227) -> ()
      }
      frame "IR Left" {
        w235 = enum16{"Monochrome", "RGB internal (RGB)"}."Monochrome" ("Color format")
        # "Mono"
        n53 = call "rs3_MemCopyRGB_IR2.vi"("Zimage pointer"=w242, "RGB  X, width"=w241, "RGB Y, height"=w240, "Color format"=w235, "error in (no error)"=w238) -> ("Output Array"=w237:u8[], "error out"=w239:errorcluster)  [unwired: 8 in, 1 out]
        n54 = local write "Color format"(w235) -> ()
      }
    }
    n55 = case shown="\"IR Left\"" w123 {
      tunnel: [w191 w197 w207 w214] -> w124
      tunnel: w122 -> [_ w194 w206 w213]
      tunnel: w121 -> [_ w193 w205 w212]
      tunnel: w120 -> [_ w195 w204 w211]
      tunnel: w125 -> [w191 w198 _ _]
      tunnel: w117 -> [w190 _ w202 w209]
      tunnel: [w190 w199 w202 w209] -> w110
      tunnel: [w189 w200 w203 w210] -> w112
      tunnel: w115 -> [w189 w200 _ _]
      tunnel: w105 -> [_ w192 _ _]
      frame "Color (ext.)", Default {
      }
      frame "Depth" {
        w196 = u16 0 items=["Y16", "Y8"] ("Image format")
        # "Depth"
        n56 = call "rs3_MemCopyUINT16_3.vi"("Image format"=w196, "Transpose"=w192, "error in (no error)"=w198, "Depth Y"=w195, "Depth X"=w193, "Zimage pointer"=w194) -> ("error out"=w197:errorcluster, "2D Array Output"=w199:sgl[][])  [unwired: 2 in, 2 out]
      }
      frame "Color (left) " {
        w201 = enum16{"Monochrome", "RGB internal (RGB)"}."RGB internal (RGB)" ("Color format")
        # "Color"
        n57 = call "rs3_MemCopyRGB_IR2.vi"("Zimage pointer"=w206, "RGB  X, width"=w205, "RGB Y, height"=w204, "Color format"=w201) -> ("Output Array"=w203:u8[], "error out"=w207:errorcluster)  [unwired: 9 in, 1 out]
        n58 = local write "Color format"(w201) -> ()
      }
      frame "IR Left" {
        w208 = enum16{"Monochrome", "RGB internal (RGB)"}."Monochrome" ("Color format")
        # "Mono"
        n59 = call "rs3_MemCopyRGB_IR2.vi"("Zimage pointer"=w213, "RGB  X, width"=w212, "RGB Y, height"=w211, "Color format"=w208) -> ("Output Array"=w210:u8[], "error out"=w214:errorcluster)  [unwired: 9 in, 1 out]
        n60 = local write "Color format"(w208) -> ()
      }
    }
    n61 = case shown="\"Color + Depth\"" "Display tab" {
      tunnel: w112 -> [_ w148 w168 _]
      tunnel: w111 -> [_ w150 w167 _]
      tunnel: w109 -> [_ w149 w166 _]
      tunnel: w110 -> [_ w147 w155 _]
      tunnel: w108 -> [_ _ w157 _]
      tunnel: w107 -> [_ _ w156 _]
      frame "Initialize", Default {
      }
      frame "Color + Depth" {
        (unwired) sgl[][] []  # Blank depthmap
        (unwired) picture bytes[33]  # Blank picture
        # "Only D415 can give color stream from left imager.\nWith other cameras monochrome stream is used."
        n62 = local read "Color format"() -> (w145:enum16{"Monochrome", "RGB internal (RGB)"})
        n63 = call "rs3_RGB_to_Picture5.vi"("RGB array"=w148, "Color format"=w145, "RGB  X, width"=w150, "RGB Y, height"=w149, "AWB"=FALSE, "White Balance"=FALSE) -> ("new picture"=→"RGB image":picture)  [unwired: 8 in, 1 out]
        "Depth map" <- w147
      }
      frame "PointCloud" {
        # "Convert color for 3D Picture format"
        # "Create x,y,z for PointCloud 3D Picture"
        n64 = for {
          tunnel: w155 -> [w171] mode=indexing
          tunnel: [w170] -> w153 mode=concatenating
          i -> [w169]
          n65 = for {
            tunnel: w171 -> [w188] mode=indexing
            tunnel: w169 -> [w187]
            tunnel: [w172] -> w170 mode=indexing
            i -> [w186]
            n66 = local read "ppx"() -> (w179:sgl)
            n67 = local read "ppy"() -> (w177:sgl)
            n68 = To Double Precision Float(number=w187) -> (double precision float=w176:dbl)
            n69 = To Double Precision Float(number=w186) -> (double precision float=w181:dbl)
            n70 = Subtract(x=w181, y=w179) -> (x-y=w180:dbl)
            n71 = Subtract(x=w176, y=w177) -> (x-y=w175:dbl)
            n72 = To Double Precision Float(number=w188) -> (double precision float=w174:dbl)
            n73 = Multiply(x=w174, y=w180) -> (x*y=w185:dbl)
            n74 = Multiply(x=w174, y=w175) -> (x*y=w182:dbl)
            n75 = local read "fx"() -> (w184:sgl)
            n76 = local read "fy"() -> (w178:sgl)
            n77 = Divide(x=w185, y=w184) -> (x/y=w183:dbl)
            n78 = Divide(x=w182, y=w178) -> (x/y=w173:dbl)
            n79 = Bundle(w183, w173, w174) -> (w172:cluster{dbl, dbl, dbl})  [unwired: 1 in]
          }
        }
        n80 = call "rs3_ExtractColor5.vi"("Manual \nWhite Balance"=FALSE ("White Balance"), "24bit Color Array"=w168, "Color format"="Color format", "Depth Y"=w166, "RGB  X"=w167, "RGB Y"=w166, "Depth X"=w167) -> ("Norm Mesh Color"=w160:T9)  [unwired: 8 in]
        n81 = call <vilib>:"Create Mesh.vi"() -> ("New Mesh Refnum"=w162:refnum<vi>)  [unwired: 10 in, 1 out]
        n82 = invoke class="SceneMesh" method="SetMeshParms"(reference=w162, "DrawMode"=T7."Points" ("Draw Mode"), "VertArray"=w153, "Indices"=w156, "ColorMode"=T6."Per Vertex" ("Color Binding Mode"), "ColorArray"=w160) -> (reference out=w163:refnum<vi>, error out=w164:errorcluster)  [unwired: 5 in, 9 out]
        n83 = invoke class="SceneObject" method="Set Drawable"(reference=w157, error in=w164, "Drawable"=w163) -> (reference out=→"3D Picture":refnum<vi>)  [unwired: 1 in, 3 out]
      }
      frame "Errors" {
      }
    }
    n84 = call "rs3 release frame.vi"("error in (no error)"=w124, "Frame"=w114) -> ("error out"=w136:errorcluster, "error"=w127:u64)  [unwired: 8 in]
    n85 = call "rs3 showError.vi"("error"=w127) -> ("Error summary"=→"release frame error":string)  [unwired: 6 in, 4 out]
    n86 = call "rs3 release frame.vi"("error in (no error)"=w136, "Frame"=w113) -> ("error out"=w135:errorcluster)  [unwired: 8 in, 1 out]
    n87 = Or(x="stop and exit", y="stop") -> (x .or. y?=w104:bool)
    "iteration" <- w139
  }
  n88 = flat-sequence {
    tunnel: [w247] -> w16
    tunnel: [w245] -> w2
    tunnel: [w243] -> _
    tunnel: [w244] -> _
    tunnel: [w244] -> _
    tunnel: [w243] -> _
    tunnel: [w243] -> _
    tunnel: w4 -> [w244]
    tunnel: w3 -> [w243]
    frame #0 {
      # "Cleate Point-Cloud Object"
      n89 = call <vilib>:"New Light.vi"("At Infinity"=TRUE) -> ("New Light Refnum"=w255:refnum<vi>)  [unwired: 2 in, 8 out]
      n90 = property class="SceneLight"(reference=w255, "Direction"=cluster{"X":sgl, "Y":sgl, "Z":sgl} {"X"=0.0, "Y"=0.0, "Z"=10000.0}, "Diffuse Color"=T12 {"Alpha"=1.0, "Blue"=1.0, "Green"=1.0, "Red"=1.0}, "atInfinity"=TRUE ("At Infinity"), "Light Number"=0, "Position"=T11 {"X"=10000.0, "Y"=0.0, "Z"=10000.0}, "Specular Color"=T10 {"Red"=1.0, "Green"=0.0, "Blue"=0.0, "Alpha"=0.0}) -> (reference out=w252:refnum<vi>)  [unwired: 1 in, 1 out]
      n91 = call-poly <vilib>:"Create Object.vi"("Name"="PointCloud Object") -> ("Scene:New Object"=w254:refnum<vi>)  [unwired: 9 in, 1 out]
      n92 = Multiply(x=w244, y=w243) -> (x*y=w246:i32)
      n93 = for {
        N: w246 -> [_]
        tunnel: [w259] -> w245 mode=indexing
        i -> [w259]
        # "indices"
      }
      n94 = invoke class="SceneObject" method="Light.Add Light"(reference=w254, "Light"=w252) -> (reference out=w247:refnum<vi>)  [unwired: 2 in, 3 out]
    }
  }
  n95 = call "rs3_close all2.vi"("Stop and Exit"=w5, "rscontext"=w6, "queue in"=w41, "error in (no error)"=w40, "device_list"=w37, "Dev in"=w21, "Sensor in"=w32) -> ("Close Error"=→"Close Error":string)  [unwired: 3 in, 1 out]
